vi "JoysticPC.vi"() -> ()   [LabVIEW 2020]
uses:
  Gamepad_Interface.ctl
  <vilib>/Platform/TimedLoop/XDataNode/timing_clust.ctl
  <vilib>/Platform/TimedLoop/XDataNode/nitl_modes.ctl
  <vilib>/Platform/TimedLoop/XDataNode/wakeup.ctl
  <vilib>/Utility/inputDevices.llb/closeJoystick.vi
  <vilib>/Platform/TimedLoop/XDataNode/XDataNode.xnode
  <vilib>/Platform/TimedLoop/XDataNode/XDNodeRunTimeDep.lvlib
panel:
  out "Gamepad_Interface":T1 {"RStick_Y" scale=-1.0..1.0; "RStick_X" scale=-1.0..1.0; "LStick_Y" scale=-1.0..1.0; "RStick_X" scale=-1.0..1.0; "RT" scale=-1.0..1.0; "LT" scale=-1.0..1.0}
  in  "STOP":bool
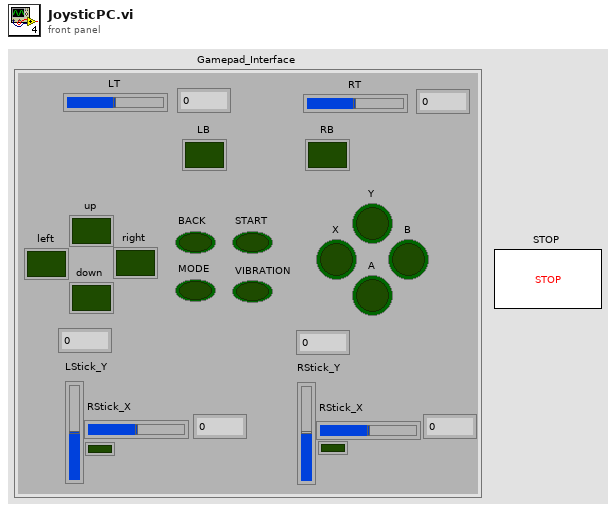
[diagram p1: front panel]
types:
  T1 = typedef "Gamepad_Interface.ctl" = cluster{"left":bool, "up":bool, "down":bool, "right":bool, "Y":bool, "X":bool, "A":bool, "B":bool, "BACK":bool, "START":bool, "MODE":bool, "VIBRATION":bool, "LB":bool, "RB":bool, "LT":dbl, "RT":dbl, "RStick_X":dbl, "LStick_Y":dbl, "RStick_X":dbl, "RStick_Y":dbl, "左杆":bool, "右杆":bool}
  T2 = cluster{"axes total":u32, "buttons total":u32, "pov total":u32, "device name":string}[]
  T3 = typedef "XDNodeRunTimeDep.lvlib/timing_clust.ctl" = cluster{"Expected End [f-1]":u64, "Actual End [f-1]":u64, "Finished Late? [f-1]":bool, "Expected End [i-1]":u64, "Actual End [i-1]":u64, "Finished Late? [i-1]":bool, "Expected Start [i]":u64, "Actual Start [i]":u64, "Expected Start [f]":u64, "Actual Start [f]":u64, "Source Name":string, "Structure Name":string, "Period":i64, "Deadline":i64, "Offset":i64, "Start":i64, "Priority":i32, "Timeout":i32, "Mode":T4, "Wakeup Reason":T5, "Error":errorcluster, "Source Type":string, "Secondary Source Type":string, "Global End Time":u64, "Global Start Time":u64, "Frame Duration":u64, "Iteration Duration":u64, "Assigned CPU":i32, "I/O Scan Engine Mode":u32}
  T4 = typedef "XDNodeRunTimeDep.lvlib/nitl_modes.ctl" = enum32{"No Change", "Process missed periods, maintain original phase", "Discard missed periods, maintain original phase", "Process missed periods, ignore original phase", "Discard missed periods, ignore original phase"}
  T5 = typedef "XDNodeRunTimeDep.lvlib/wakeup.ctl" = enum32{"Normal", "Aborted", "Asynchronous wakeup", "Timing source error", "Timed loop error", "Timeout"}
  T6 = typedef "joystick.ctl" = cluster{"left":bool, "up":bool, "dowm":bool, "right":bool, "Y":bool, "X":bool, "A":bool, "B":bool, "BACK":bool, "START":bool, "MODE":bool, "VIBRATION":bool, "LB":bool, "RB":bool, "LT":dbl, "RT":dbl, "左横杆":dbl, "左竖杆":dbl, "右横杆":dbl, "右竖杆":dbl, "左杆":bool, "右杆":bool}
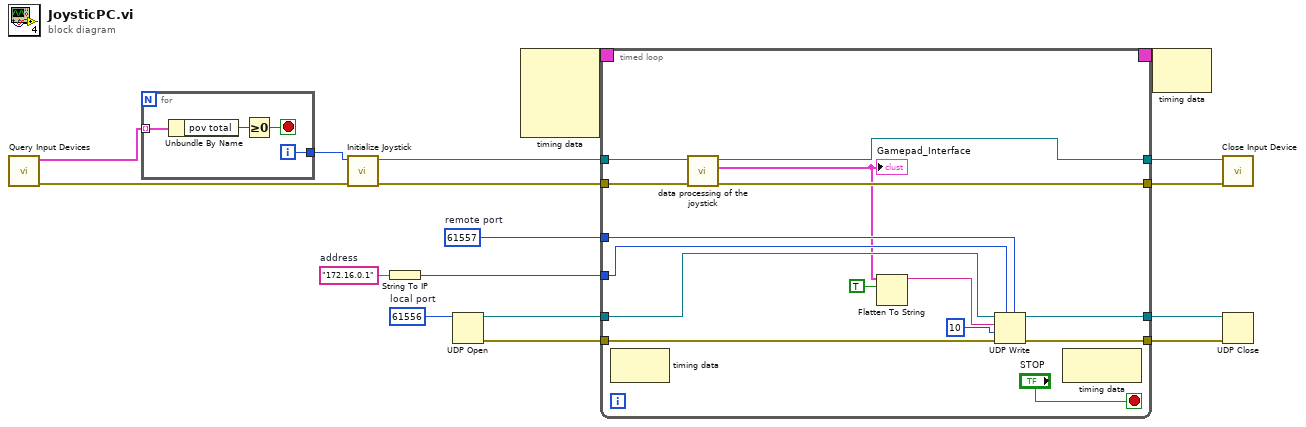
[diagram p0: block diagram]
diagram:
  w6 = "172.16.0.1"  # address
  w10 = u16 61557  # remote port
  w3 = u16 61556  # local port
  n1 = call <vilib>:"Query Input Devices.vi"() -> ("error out"=w15:errorcluster, "joystick info"=w17:T2)  [unwired: 8 in, 2 out]
  n2 = for {
    tunnel: w17 -> [w21] mode=indexing
    tunnel: [w18] -> w16
    i -> [w18]
    stop <- w20 stop-if-true
    n3 = Unbundle By Name(w21) -> ("pov total"=w19:u32)
    n4 = Greater Or Equal To 0?(x=w19) -> (x >= 0?=w20:bool)
  }
  n5 = call <vilib>:"Initialize Joystick.vi"("error in (no error)"=w15, "device index"=w16) -> ("error out"=w13:errorcluster, "device ID"=w14:refnum<k1>)  [unwired: 8 in]
  n6 = String To IP(1:w6) -> (0:w7:u32)
  n7 = UDP Open(11:w3) -> (port=w5:refnum<k16>, 0:w4:errorcluster)  [unwired: 4 in, 1 out]
  n8 = node-c288() -> (w2:T3)  [unwired: 4 in]
  n9 = timed-loop {
    tunnel: w14 -> [w36]
    tunnel: [w34] -> w11
    tunnel: w13 -> [w35]
    tunnel: [w32] -> w12
    tunnel: w10 -> [w25]
    tunnel: w5 -> [w31]
    tunnel: [w30] -> w9
    tunnel: [w29] -> w8
    tunnel: w4 -> [w28]
    tunnel: w7 -> [w27]
    timing: w2 -> [_]
    timing-out: [_] -> w1
    stop <- "STOP" stop-if-true
    n10 = node-c288() -> ()  [unwired: 1 in, 1 out]
    n11 = call <vilib>:"data processing of the joystick.vi"("错误输入（无错误）"=w35, "引用句柄输入"=w36) -> ("错误输出"=w32:errorcluster, "joystick"=w24:T6, "引用句柄输出"=w34:refnum<k1>)  [unwired: 7 in]
    "Gamepad_Interface" <- w24
    n12 = Flatten To String(anything=w24, prepend array or string size? (T)=TRUE) -> (data string=w26:string)  [unwired: 2 in, 2 out]
    n13 = UDP Write(address=w27, port or service name=w25, connection ID=w31, data in=w26, 8:w28, 9:10 ("timeout ms (25000)")) -> (error out=w29:errorcluster, 3:w30:refnum<k16>)
    n14 = node-c288() -> ()  [unwired: 1 in, 1 out]
  }
  n15 = node-c288(w1) -> ()  [unwired: 1 out]
  n16 = call-poly <vilib>:"Close Input Device.vi"("error in (no error)"=w12, "device ID"=w11) -> ()  [unwired: 8 in, 1 out]
  n17 = UDP Close(connection ID=w9, 8:w8) -> ()  [unwired: 2 out]
